vi "LIN Init.vi"(9 "pConfig":T1, 10 "LINIndex":u8, 11 "DevHandle":i32) -> (1 "pConfig out":T1, 3 "function return":i32)   [LabVIEW 2010, in "usb2lin.lvlib"]
doc: "int WINAPI LIN_Init(int DevHandle,unsigned char LINIndex,LIN_CONFIG *pConfig);"
uses:
  usb2lin.lvlib
  USB2XXX/trunk/USB2XXX/USB2XXX/vs2010/Release/USB2XXX.dll
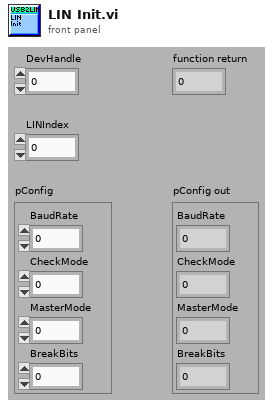
[diagram p1: front panel]
types:
  T1 = cluster{"BaudRate":u32, "CheckMode":u8, "MasterMode":u8, "BreakBits":u8}
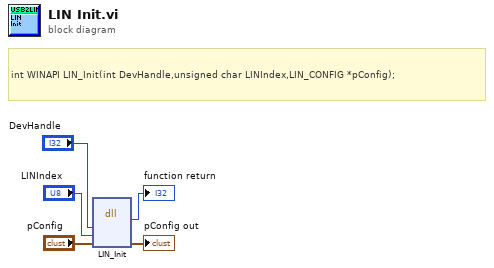
[diagram p0: block diagram]
diagram:
  # "int WINAPI LIN_Init(int DevHandle,unsigned char LINIndex,LIN_CONFIG *pConfig);"
  n1 = dll-call lib="E:/OtherWork/STM32/USB2XXX/trunk/USB2XXX/USB2XXX/vs2010/Release/USB2XXX.*" fn="LIN_Init"("DevHandle"="DevHandle", "LINIndex"="LINIndex", "pConfig"="pConfig") -> (→"function return":i32, "pConfig"=→"pConfig out":T1)  [unwired: 5 in, 2 out]
